vi "InjA-Image-RT.vi"() -> ()   [LabVIEW 2016]
uses:
  Controls/Cryo Readback.ctl
  Controls/Aperture states.ctl
  Controls/Faraday cup states.ctl
  Controls/GV states.ctl
  Controls/GP307 cluster.ctl
  <vilib>/userdefined/High Color/nirio_resource_hc.ctl
  PRIMELab-2017/Control/Common-Control/Glassman Control.ctl
  <vilib>/FPGAPlugInAG/cRIO-9074/niLvFpga_Open_cRIO-9074.vi
  <vilib>/Utility/error.llb/Error Cluster From Error Code.vi
  <vilib>/rvi/errors/niLvFpgaAdjustHostInterfaceError.vi
  <vilib>/functionblocks/Control/PID/PID.vi
  <vilib>/rvi/interface/nirviOpenFPGA/nirviOpenFPGA.xnode
  FPGA Bitfiles/Controlsoftware2_FPGATarget_InjFPGA_-aTnSXeY2bA.lvbitx
  InjA-Image-FPGA.vi
  <vilib>/rvi/interface/nirviReadWriteControl/nirviReadWriteControl.xnode
  <vilib>/functionblocks/FB Core/FB Core.xnode
  <vilib>/functionblocks/FB Property/FB Overlay DBL.ctl
  <vilib>/functionblocks/NI_FunctionBlock Libraries.lvlib
  NiFpgaLv.dll
  <vilib>/NI_Real-Time Target Support.lvlib
panel:
  in  "Tab Control":T1(tab)
  out "X-I":fxp<+/-,16,5>=1.28955078125
  out "X- V":fxp<+/-,16,5>=5.3388671875
  out "X+ I":fxp<+/-,16,5>=1.1064453125
  out "X+ V":fxp<+/-,16,5>=4.63671875
  out "Y+ V":fxp<+/-,16,5>=4.380859375
  out "Y+I":fxp<+/-,16,5>=1.068359375
  out "Y-V":fxp<+/-,16,5>=5.595703125
  out "Y-I":fxp<+/-,16,5>=1.36572265625
  out "Pre-acc V":fxp<+/-,16,5>=8.2509765625
  out "Pre-acc I":fxp<+/-,16,5>=2.544921875
  out "Einzel V":fxp<+/-,16,5>=7.4140625
  out "Einzel I":fxp<+/-,16,5>=1.6787109375
  out "X- Steerer Voltage Set":dbl
  out "X- Steerer HV Enable":bool
  out "X+ Steerer HV Enable":bool
  out "X+ Steerer Voltage Set":dbl
  out "Y- Steerer voltage set":dbl
  out "Y- Steerer HV Enable":bool
  out "Y+ Steerer HV Enable":bool
  out "Y+ Steerer voltage set":dbl
  out "Pre-Acc V set":dbl
  out "Pre-Acc HV Enable":bool
  out "Einzel HV Enable":bool
  out "Einzel V set":dbl
  in  "output low - injector":dbl
  in  "output high - injector":dbl=190.0
  out "Injector mag field set":dbl
  out "Injector mag field read 2":u8[](array[numeric])
  out "Injector mag field read":dbl
  out "Injector mag ps command":u8[](array[numeric])
  in  "derivative time (Td, min) - injector":dbl=0.01
  in  "integral time (Ti, min) - injector":dbl=0.01
  in  "proportional gain (Kc) - injector":dbl=10.0
  out "Injector mag command string":string
  out "Cryo Readback":T2
  out "Status":string
  out "On-time":string
  out "1st Stage Temp":string
  out "2nd Stage Temp":string
  out "Time since re-purge":string
  out "LowEnd Waist Vac Interlock":bool
  out "LowEnd Waist Vac Interlock bypass":bool
  out "Vac Interlock":bool
  out "Time since repurge":u8[](array[numeric])
  out "2nd stage temp":u8[](array[numeric])
  out "Cryo 1st stage temp":u8[](array[numeric])
  out "Cryo On-time":u8[](array[numeric])
  out "Cryo status":u8[](array[numeric])
  out "InjA Image Interlock bypass":bool
  out "Convectron 2":u8[](array[numeric])
  out "Ion Gauge 2":u8[](array[numeric])
  out "InjA Image Ion Gauge 1":dbl
  out "InjA Image Vac Cluster":T3
  out "InjA Image Convectron 1":dbl
  out "Convectron 1":u8[](array[numeric])
  out "Ion Gauge 1":u8[](array[numeric])
  out "Injector A Vac Interlock":bool
  out "Injector A Vac Interlock Bypass":bool
  out "Inj Image Aperture actuator":bool
  out "Inj Image FC actuator":bool
  out "Cryo Pump GV actuator":bool
  out "Beamline GV actuator":bool
  out "Inj Image Image  Aperture Position 2":T4
  out "Inj Image Image  Aperture Position":cluster{"IN sensor":bool, "OUT sensor":bool}
  out "Inj Image FC Status":T5
  out "Inj Image FC Position":cluster{"IN sensor":bool, "OUT sensor":bool}
  out "Beamline GV status":T6
  out "Beamline GV Position":T7
  out "Cryo Pump GV status":T6
  out "Cryo Pump GV Position":T7
  out "HV control loop error":errorcluster
  out "HV Readback loop error":errorcluster
  out "Injector Magnet error":errorcluster
  out "Cryo loop error":errorcluster
  out "GV Interlock loop error":errorcluster
  out "Acuator-Sensor loop error":errorcluster
  out "Vac cluster loop error":errorcluster
  out "Error Reporter":errorcluster
  in  "error in":errorcluster
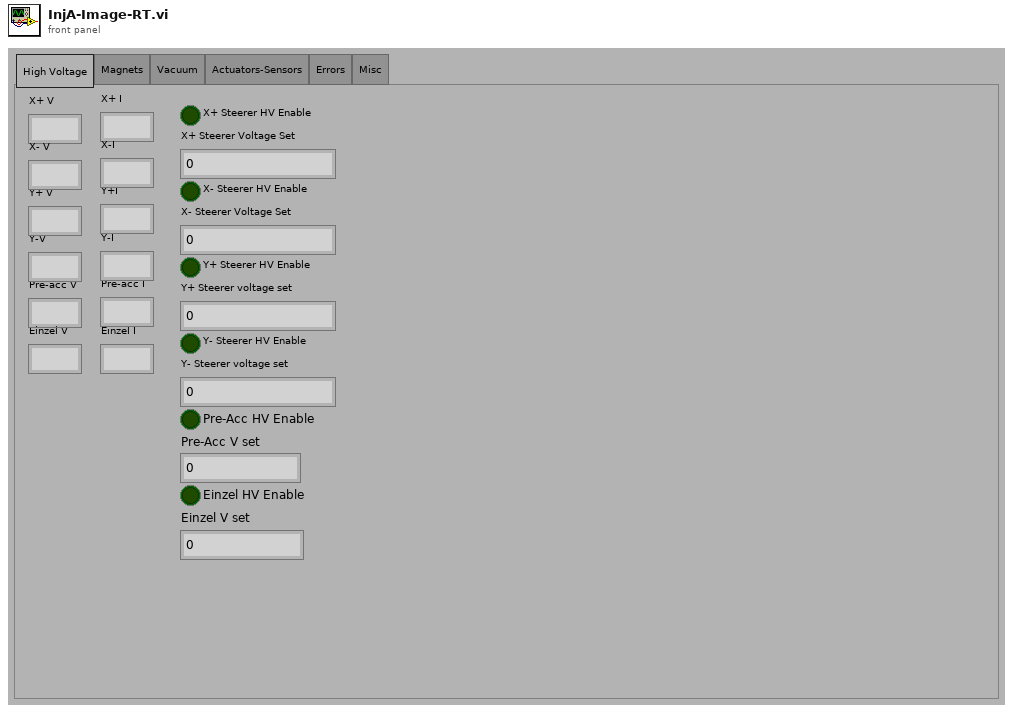
[diagram p1: front panel]
types:
  T1 = enum32{"High Voltage", "Magnets", "Vacuum", "Actuators-Sensors", "Errors", "Misc"}
  T2 = typedef "Cryo Readback.ctl" = cluster{"Status":string, "On-time":string, "1st Stage Temp":string, "2nd Stage Temp":string, "Time since re-purge":string}
  T3 = typedef "GP307 cluster.ctl" = cluster{"Ion gauge 1":string, "Convectron  Gauge 1 ":string, "Ion Gauge 2":string, "Convectrom Gauge 2":string}
  T4 = typedef "Aperture states.ctl" = enum16{"Aperture status unclear", "Aperture in", "Aperture out"}
  T5 = typedef "Faraday cup states.ctl" = enum16{"FC status unclear", "FC in", "FC out"}
  T6 = typedef "GV states.ctl" = enum16{"status unclear", "closed", "open"}
  T7 = cluster{"OPEN sensor":bool, "Closed sensor":bool}
  T8 = typedef "nirio_resource_hc.ctl" = tag
  T9 = cluster{"Stable 1":dbl, "Rare":dbl, "Stable 2":dbl}
  T10 = typedef "Glassman Control.ctl" = cluster{"V-program":fxp<+/-,16,5>, "HV Enable":bool}
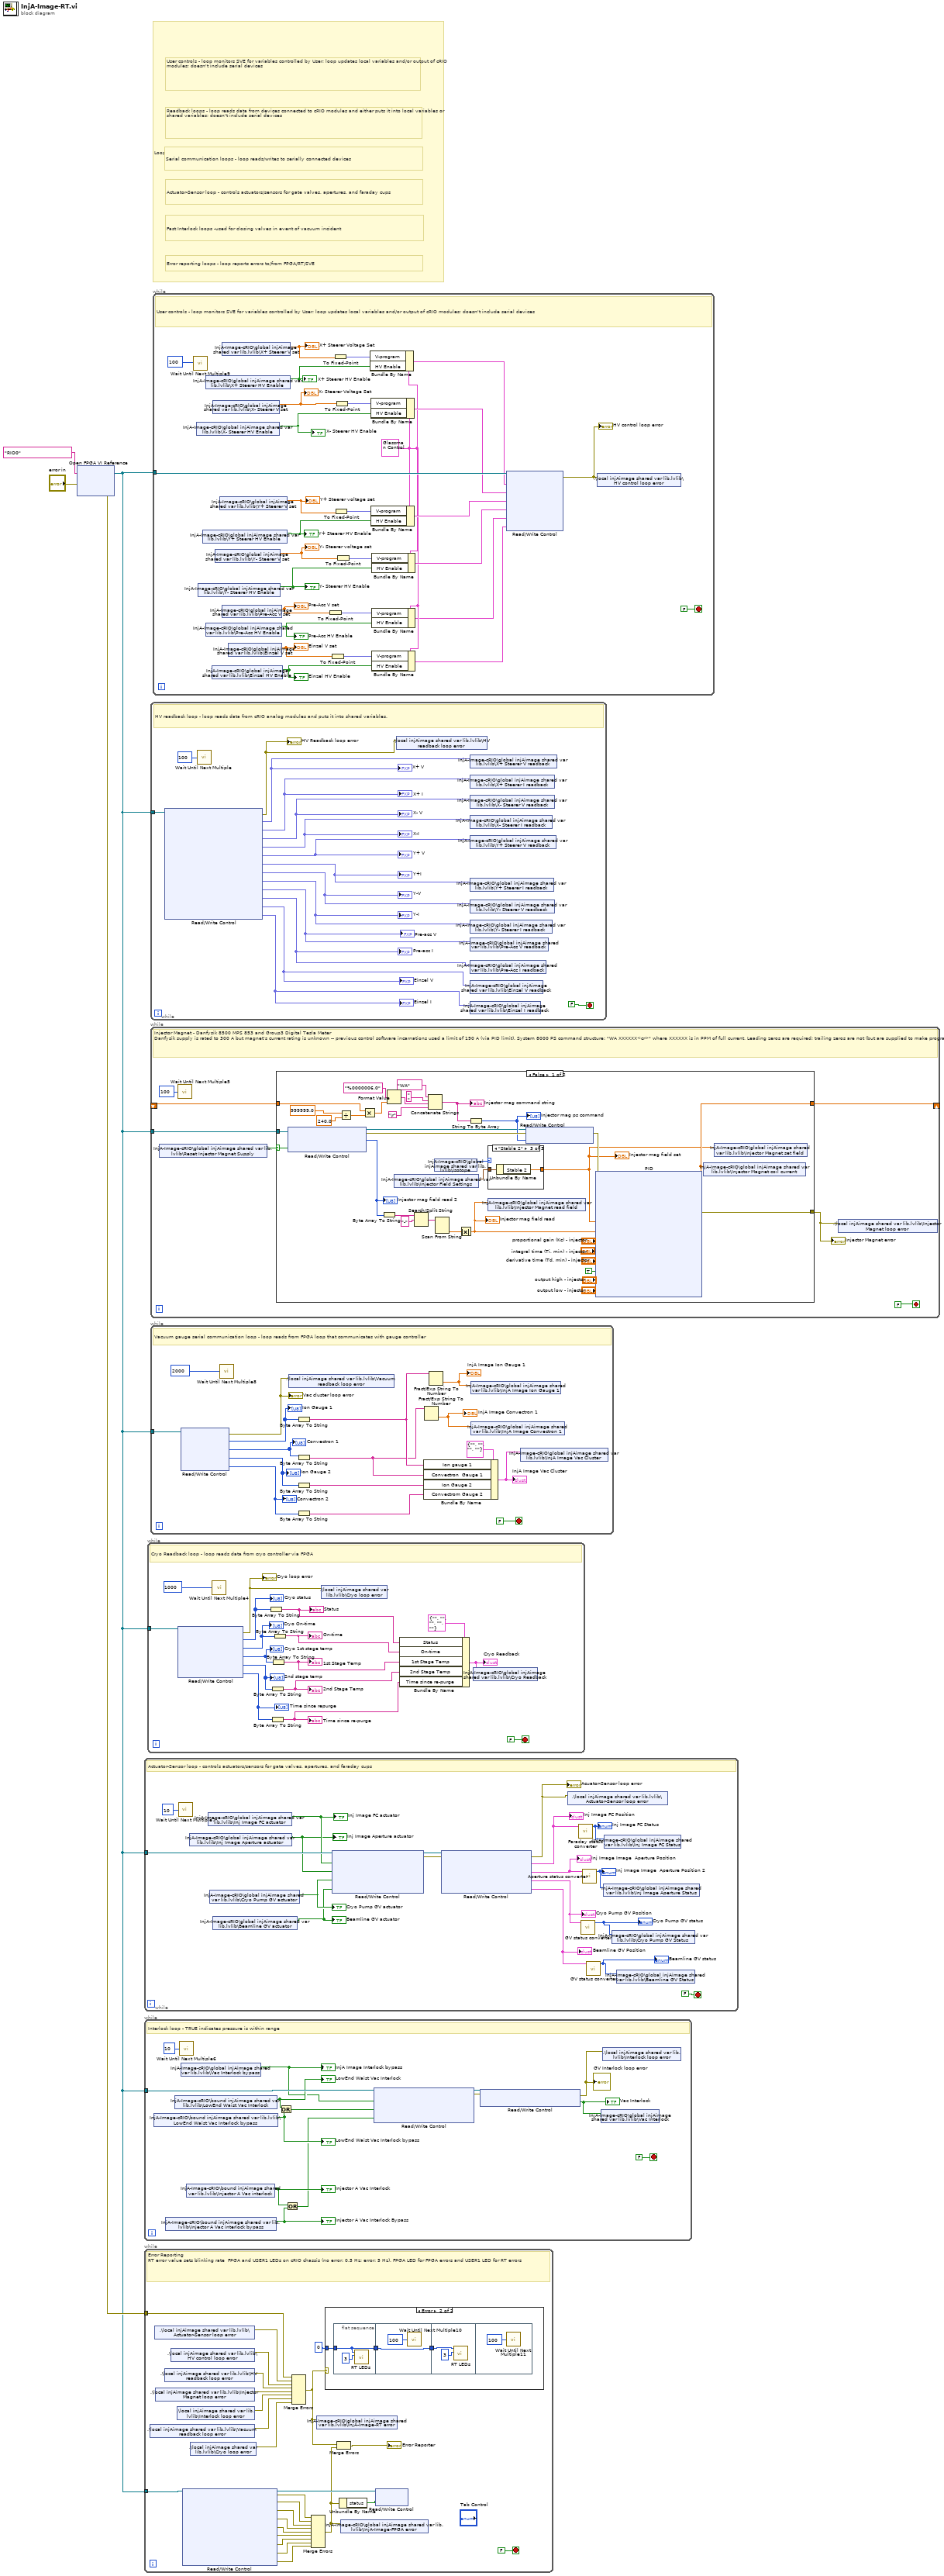
[diagram p0: block diagram]
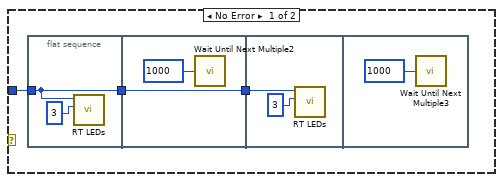
[diagram p2: hidden frame]
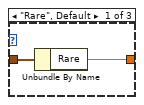
[diagram p3: hidden frame]
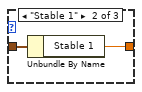
[diagram p4: hidden frame]
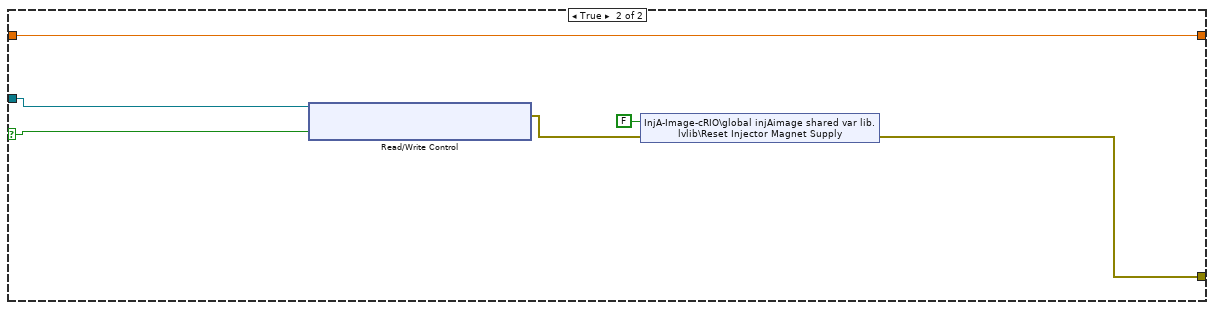
[diagram p5: hidden frame]
diagram:
  # "Serial communication loops - loop reads/writes to serially connected devices"
  # "Actuator-Sensor loop - controls actuators/sensors for gate valves, apertures, and faraday cups"
  # "Fast Interlock loops -used for closing valves in event of vacuum incident"
  # "Error reporting loops - loop reports errors to/from FPGA/RT/SVE"
  # "Readback loops - loop reads data from devices connected to cRIO modules and either puts it into local variables or shared variables; doesn't include serial devices"
  # "User controls - loop monitors SVE for variables controlled by User; loop updates local variables and/or output of cRIO modules; doesn't include serial devices"
  # "Loop legend - loops are color coded by responsibility"
  n1 = xnode "Open FPGA VI Reference"("error in"="error in", "resource name"=T8 "RIO0") -> ("FPGA VI Reference Out"=w1:refnum<k20>, "error out"=w2:errorcluster)
  n2 = while {
    tunnel: w1 -> [w22]
    stop <- FALSE stop-if-true
    # "Actuator-Sensor loop - controls actuators/sensors for gate valves, apertures, and faraday cups"
    n3 = call "Wait Until Next Multiple7"("Count(mSec)"=u32 10) -> ()  [unwired: 1 out]
    n4 = shared-variable "InjA-Image-cRIO\\global injAimage shared var lib.lvlib\\Inj Image Aperture actuator"() -> (w8:bool)  [unwired: 1 in, 1 out]
    "Inj Image Aperture actuator" <- w8
    n5 = shared-variable "InjA-Image-cRIO\\global injAimage shared var lib.lvlib\\Inj Image FC actuator"() -> (w9:bool)  [unwired: 1 in, 1 out]
    "Inj Image FC actuator" <- w9
    n6 = shared-variable "InjA-Image-cRIO\\global injAimage shared var lib.lvlib\\Cryo Pump GV actuator"() -> (w11:bool)  [unwired: 1 in, 1 out]
    "Cryo Pump GV actuator" <- w11
    n7 = shared-variable "InjA-Image-cRIO\\global injAimage shared var lib.lvlib\\Beamline GV actuator"() -> (w10:bool)  [unwired: 1 in, 1 out]
    "Beamline GV actuator" <- w10
    n8 = xnode "Read/Write Control"("FPGA VI Reference In"=w22, "Inj Image FC Actuator"=w9, "Inj Image Aperture Actuator"=w8, "Cryo Pump GV Actuator"=w11, "Beamline GV Actuator"=w10) -> ("FPGA VI Reference Out"=w20:refnum<k20>, "error out"=w18:errorcluster)  [unwired: 1 in]
    n9 = xnode "Read/Write Control"("FPGA VI Reference In"=w20, "error in"=w18) -> ("error out"=w12:errorcluster, "Inj Image FC Position"=w14:cluster{"IN sensor":bool, "OUT sensor":bool}, "Inj Image Aperture Position"=w13:cluster{"IN sensor":bool, "OUT sensor":bool}, "Cryo Pump GV Status"=w17:T7, "Beamline GV Status"=w16:T7)  [unwired: 1 out]
    "Cryo Pump GV Position" <- w17
    "Beamline GV Position" <- w16
    "Inj Image FC Position" <- w14
    "Inj Image Image  Aperture Position" <- w13
    "Acuator-Sensor loop error" <- w12
    n10 = shared-variable ".\\local injAimage shared var lib.lvlib\\Actuator-Sensor loop error"(w12) -> ()  [unwired: 1 in, 1 out]
    n11 = call "Faraday status converter.vi"("FC Position"=w14) -> ("FC Status"=w15:T5)  [unwired: 10 in]
    "Inj Image FC Status" <- w15
    n12 = call "GV status converter.vi"("Gate Valve"=w17) -> ("GV Status"=w6:T6)  [unwired: 10 in]
    "Cryo Pump GV status" <- w6
    n13 = call "Aperture status converter.vi"("Aperture Position"=w13) -> ("Aperture Status"=w5:T4)  [unwired: 10 in]
    "Inj Image Image  Aperture Position 2" <- w5
    n14 = call "GV status converter.vi"("Gate Valve"=w16) -> ("GV Status"=w7:T6)  [unwired: 10 in]
    "Beamline GV status" <- w7
    n15 = shared-variable "InjA-Image-cRIO\\global injAimage shared var lib.lvlib\\Inj Image Aperture Status"(w5) -> ()  [unwired: 1 in, 1 out]
    n16 = shared-variable "InjA-Image-cRIO\\global injAimage shared var lib.lvlib\\Inj Image FC Status"(w15) -> ()  [unwired: 1 in, 1 out]
    n17 = shared-variable "InjA-Image-cRIO\\global injAimage shared var lib.lvlib\\Cryo Pump GV Status"(w6) -> ()  [unwired: 1 in, 1 out]
    n18 = shared-variable "InjA-Image-cRIO\\global injAimage shared var lib.lvlib\\Beamline GV Status"(w7) -> ()  [unwired: 1 in, 1 out]
  }
  n19 = while {
    tunnel: w1 -> [w36]
    stop <- FALSE stop-if-true
    # "Interlock loop - TRUE indicates pressure is within range"
    n20 = shared-variable "InjA-Image-cRIO\\bound injAimage shared var lib.lvlib\\LowEnd Waist Vac Interlock bypass"() -> (w30:bool)  [unwired: 1 in, 1 out]
    "LowEnd Waist Vac Interlock bypass" <- w30
    n21 = shared-variable "InjA-Image-cRIO\\bound injAimage shared var lib.lvlib\\Injector A Vac interlock bypass"() -> (w25:bool)  [unwired: 1 in, 1 out]
    "Injector A Vac Interlock Bypass" <- w25
    n22 = shared-variable "InjA-Image-cRIO\\bound injAimage shared var lib.lvlib\\LowEnd Waist Vac Interlock"() -> (w28:bool)  [unwired: 1 in, 1 out]
    "LowEnd Waist Vac Interlock" <- w28
    n23 = call "Wait Until Next Multiple6"("Count(mSec)"=u32 10) -> ()  [unwired: 1 out]
    n24 = shared-variable "InjA-Image-cRIO\\global injAimage shared var lib.lvlib\\Vac Interlock bypass"() -> (w23:bool)  [unwired: 1 in, 1 out]
    "InjA Image Interlock bypass" <- w23
    n25 = shared-variable "InjA-Image-cRIO\\bound injAimage shared var lib.lvlib\\Injector A Vac interlock"() -> (w26:bool)  [unwired: 1 in, 1 out]
    "Injector A Vac Interlock" <- w26
    n26 = Or(x=w28, y=w30) -> (x .or. y?=w29:bool)
    n27 = Or(x=w26, y=w25) -> (x .or. y?=w24:bool)
    n28 = xnode "Read/Write Control"("FPGA VI Reference In"=w36, "Vac Interlock Bypass"=w23, "LowEnd Waist Vac Interlock"=w29, "InjectorA Vac Interlock"=w24) -> ("FPGA VI Reference Out"=w35:refnum<k20>, "error out"=w34:errorcluster)  [unwired: 1 in]
    n29 = xnode "Read/Write Control"("FPGA VI Reference In"=w35, "error in"=w34) -> ("error out"=w33:errorcluster, "Vac Interlock"=w27:bool)  [unwired: 1 out]
    "GV Interlock loop error" <- w33
    "Vac Interlock" <- w27
    n30 = shared-variable "InjA-Image-cRIO\\global injAimage shared var lib.lvlib\\Vac Interlock"(w27) -> ()  [unwired: 1 in, 1 out]
    n31 = shared-variable ".\\local injAimage shared var lib.lvlib\\Interlock loop error"(w33) -> ()  [unwired: 1 in, 1 out]
  }
  n32 = while {
    tunnel: w1 -> [w60]
    tunnel: w2 -> [w44]
    stop <- FALSE stop-if-true
    # "Error Reporting\nRT error value sets blinking rate  FPGA and USER1 LEDs on cRIO chassis (no error: 0.5 Hz; error: 5 Hz). FPGA LED for FPGA errors and USER1 LED for RT errors"
    n33 = shared-variable ".\\local injAimage shared var lib.lvlib\\Vacuum readback loop error"() -> (w46:errorcluster)  [unwired: 1 in, 1 out]
    n34 = shared-variable ".\\local injAimage shared var lib.lvlib\\Actuator-Sensor loop error"() -> (w43:errorcluster)  [unwired: 1 in, 1 out]
    n35 = shared-variable ".\\local injAimage shared var lib.lvlib\\Injector Magnet loop error"() -> (w48:errorcluster)  [unwired: 1 in, 1 out]
    n36 = shared-variable ".\\local injAimage shared var lib.lvlib\\HV readback loop error"() -> (w49:errorcluster)  [unwired: 1 in, 1 out]
    n37 = shared-variable ".\\local injAimage shared var lib.lvlib\\HV control loop error"() -> (w42:errorcluster)  [unwired: 1 in, 1 out]
    n38 = shared-variable ".\\local injAimage shared var lib.lvlib\\Interlock loop error"() -> (w47:errorcluster)  [unwired: 1 in, 1 out]
    n39 = xnode "Read/Write Control"("FPGA VI Reference In"=w60) -> ("FPGA VI Reference Out"=w59:refnum<k20>, "error out"=w37:errorcluster, "GV Interlock loop error"=w58:errorcluster, "Actuator-Sensor Loop error"=w57:errorcluster, "Injector Hall Probe error"=w56:errorcluster, "Injector Magnet control error"=w55:errorcluster, "Vac readback loop error"=w54:errorcluster, "HV control loop error"=w53:errorcluster, "Cryo pump error"=w51:errorcluster, "HV Readback loop"=w50:errorcluster)  [unwired: 1 in]
    n40 = shared-variable ".\\local injAimage shared var lib.lvlib\\Cryo loop error"() -> (w45:errorcluster)  [unwired: 1 in, 1 out]
    n41 = Merge Errors(w44, w43, w42, w49, w48, w47, w46, w45) -> (w38:errorcluster)
    n42 = Merge Errors(w37, w58, w57, w56, w55, w54, w53, w51, w50) -> (w40:errorcluster)
    n43 = shared-variable "InjA-Image-cRIO\\global injAimage shared var lib.lvlib\\InjA-Image-RT error"(w38) -> ()  [unwired: 1 in, 1 out]
    n44 = case shown="Error" w38 {
      tunnel: 0 -> [w64 w72]
      frame No Error {
        n45 = flat-sequence {
          tunnel: w64 -> [w65]
          tunnel: [w65] -> w62
          tunnel: [w67] -> w63
          tunnel: w62 -> [w67]
          tunnel: w63 -> [w69]
          frame #0 {
            n46 = call <vilib>:"RT LEDs.vi"("State"=3, "LED Num"=w65) -> ()  [unwired: 4 in, 2 out]
          }
          frame #1 {
            n47 = call "Wait Until Next Multiple2"("Count(mSec)"=u16 1000) -> ()  [unwired: 1 out]
          }
          frame #2 {
            n48 = call <vilib>:"RT LEDs.vi"("State"=3, "LED Num"=w69) -> ()  [unwired: 4 in, 2 out]
          }
          frame #3 {
            n49 = call "Wait Until Next Multiple3"("Count(mSec)"=u16 1000) -> ()  [unwired: 1 out]
          }
        }
      }
      frame Error {
        n50 = flat-sequence {
          tunnel: [w75] -> w74
          tunnel: w72 -> [w75]
          tunnel: w74 -> [w77]
          tunnel: [w77] -> w73
          tunnel: w73 -> [w79]
          frame #0 {
            n51 = call <vilib>:"RT LEDs.vi"("State"=3, "LED Num"=w75) -> ()  [unwired: 4 in, 2 out]
          }
          frame #1 {
            n52 = call "Wait Until Next Multiple10"("Count(mSec)"=u16 100) -> ()  [unwired: 1 out]
          }
          frame #2 {
            n53 = call <vilib>:"RT LEDs.vi"("State"=3, "LED Num"=w79) -> ()  [unwired: 4 in, 2 out]
          }
          frame #3 {
            n54 = call "Wait Until Next Multiple11"("Count(mSec)"=u16 100) -> ()  [unwired: 1 out]
          }
        }
      }
    }
    n55 = Merge Errors(w38, w40) -> (→"Error Reporter":errorcluster)
    n56 = Unbundle By Name(w40) -> ("status"=w61:bool)
    n57 = shared-variable "InjA-Image-cRIO\\global injAimage shared var lib.lvlib\\InjA-Image-FPGA error"(w40) -> ()  [unwired: 1 in, 1 out]
    n58 = xnode "Read/Write Control"("FPGA VI Reference In"=w59, "RT error"=w61) -> ()  [unwired: 1 in, 2 out]
  }
  n59 = while {
    tunnel: w1 -> [w96]
    stop <- FALSE stop-if-true
    # "Cryo Readback loop - loop reads data from cryo controller via FPGA"
    n60 = xnode "Read/Write Control"("FPGA VI Reference In"=w96) -> ("error out"=w82:errorcluster, "Cryo status"=w93:u8[], "Cryo On-time"=w94:u8[], "1st stage temp"=w95:u8[], "2nd stage temp"=w92:u8[], "Time since repurge"=w91:u8[])  [unwired: 1 in, 1 out]
    "Cryo status" <- w93
    "Cryo On-time" <- w94
    "Cryo 1st stage temp" <- w95
    "Cryo loop error" <- w82
    "2nd stage temp" <- w92
    "Time since repurge" <- w91
    n61 = call "Wait Until Next Multiple4"("Count(mSec)"=u32 1000 ("millisecond multiple")) -> ()  [unwired: 1 out]
    n62 = Byte Array To String(unsigned byte array=w93) -> (string=w87:string)
    "Status" <- w87
    n63 = Byte Array To String(unsigned byte array=w92) -> (string=w84:string)
    "2nd Stage Temp" <- w84
    n64 = Byte Array To String(unsigned byte array=w91) -> (string=w83:string)
    "Time since re-purge" <- w83
    n65 = Byte Array To String(unsigned byte array=w95) -> (string=w85:string)
    "1st Stage Temp" <- w85
    n66 = Byte Array To String(unsigned byte array=w94) -> (string=w86:string)
    "On-time" <- w86
    n67 = shared-variable ".\\local injAimage shared var lib.lvlib\\Cryo loop error"(w82) -> ()  [unwired: 1 in, 1 out]
    n68 = Bundle By Name(cluster=T2 {"Status"="", "On-time"="", "1st Stage Temp"="", "2nd Stage Temp"="", "Time since re-purge"=""} ("Cryo Readback"), "Status"=w87, "On-time"=w86, "1st Stage Temp"=w85, "2nd Stage Temp"=w84, "Time since re-purge"=w83) -> (w89:T2)
    "Cryo Readback" <- w89
    n69 = shared-variable "InjA-Image-cRIO\\global injAimage shared var lib.lvlib\\Cryo Readback"(w89) -> ()  [unwired: 1 in, 1 out]
  }
  n70 = while {
    shift-right: [w100] -> _
    shift-left: _ -> [w102]
    tunnel: w1 -> [w103]
    stop <- FALSE stop-if-true
    # "Injector Magnet - Danfysik 8500 MPS 853 and Group3 Digital Tesla Meter\nDanfysik supply is rated to 300 A but magnet's current rating is unknown -- previous control software incarnations used a limit of 190 A (via PID limit). System 8000 PS command structure: \"WA XXXXXX<cr>\" where XXXXXX is in PPM of full current. Leading zeros are required; trailing zeros are not (but are supplied to make programming easier)"
    n71 = shared-variable "InjA-Image-cRIO\\global injAimage shared var lib.lvlib\\Reset Injector Magnet Supply"() -> (w99:bool)  [unwired: 1 in, 1 out]
    n72 = call "Wait Until Next Multiple5"("Count(mSec)"=u32 100 ("millisecond multiple")) -> ()  [unwired: 1 out]
    n73 = case shown="False" w99 {
      selector: w99 -> [w110 w214]
      tunnel: w103 -> [w125 w216]
      tunnel: w102 -> [w121 w215]
      tunnel: [w111 w215] -> w100
      tunnel: [w109 w211] -> w98
      frame False {
        n74 = xnode "Read/Write Control"("FPGA VI Reference In"=w125, "Inj Magnet Reset"=w110) -> ("FPGA VI Reference Out"=w119:refnum<k20>, "error out"=w124:errorcluster, "Injector Mag Field read"=w120:u8[])  [unwired: 1 in]
        "Injector mag field read 2" <- w120
        n75 = Divide(x=999999.0 ("y"), y=240.0) -> (x/y=w113:dbl)
        n76 = Multiply(x=w121, y=w113) -> (x*y=w134:dbl)
        n77 = Byte Array To String(unsigned byte array=w120) -> (string=w131:string)
        n78 = Format Value(format string="%0000006.0", value (0)=w134) -> (output string=w137:string)  [unwired: 1 out]
        n79 = shared-variable "InjA-Image-cRIO\\global injAimage shared var lib.lvlib\\Injector Field Settings"() -> (w105:T9)  [unwired: 1 in, 1 out]
        n80 = Search/Split String(string=w131, search string/char (-)="-") -> (match + rest of string=w122:string)  [unwired: 3 out]
        n81 = Concatenate Strings("WA", " ", w137, "\r") -> (w138:string)
        "Injector mag command string" <- w138
        n82 = shared-variable "InjA-Image-cRIO\\global injAimage shared var lib.lvlib\\Isotope"() -> (w107:enum16{"Rare", "Stable 1", "Stable 2"})  [unwired: 1 in, 1 out]
        n83 = Scan From String(input string=w122) -> (output 1=w130:dbl)  [unwired: 3 in, 4 out]
        n84 = Absolute Value(x=w130) -> (abs(x)=w108:dbl)
        "Injector mag field read" <- w108
        n85 = String To Byte Array(string=w138) -> (unsigned byte array=w123:u8[])
        "Injector mag ps command" <- w123
        n86 = case shown="\"Stable 2\"" w107 {
          tunnel: w105 -> [w139 w142 w144]
          tunnel: [w140 w141 w143] -> w106
          frame "Rare", Default {
            n87 = Unbundle By Name(w139) -> ("Rare"=w140:dbl)
          }
          frame "Stable 1" {
            n88 = Unbundle By Name(w142) -> ("Stable 1"=w141:dbl)
          }
          frame "Stable 2" {
            n89 = Unbundle By Name(w144) -> ("Stable 2"=w143:dbl)
          }
        }
        "Injector mag field set" <- w106
        n90 = shared-variable "InjA-Image-cRIO\\global injAimage shared var lib.lvlib\\Injector Magnet read field"(w108) -> ()  [unwired: 1 in, 1 out]
        n91 = xnode "Read/Write Control"("FPGA VI Reference In"=w119, "error in"=w124, "Injector Magnet Set"=w123) -> ("error out"=w118:errorcluster)  [unwired: 1 out]
        n92 = xnode "PID"("error in"=w118, "setpoint"=w106, "process variable"=w108, "proportional gain (Kc)"="proportional gain (Kc) - injector", "integral time (Ti, min)"="integral time (Ti, min) - injector", "derivative time (Td, min)"="derivative time (Td, min) - injector", "auto? (T)"=TRUE, "output high"="output high - injector", "output low"="output low - injector") -> ("error out"=w109:errorcluster, "output"=w111:dbl)
        n93 = shared-variable "InjA-Image-cRIO\\global injAimage shared var lib.lvlib\\Injector Magnet coil current"(w111) -> ()  [unwired: 1 in, 1 out]
        n94 = shared-variable "InjA-Image-cRIO\\global injAimage shared var lib.lvlib\\Injector Magnet set field"(w106) -> ()  [unwired: 1 in, 1 out]
      }
      frame True {
        n95 = xnode "Read/Write Control"("FPGA VI Reference In"=w216, "Inj Magnet Reset"=w214) -> ("error out"=w212:errorcluster)  [unwired: 1 in, 1 out]
        n96 = shared-variable "InjA-Image-cRIO\\global injAimage shared var lib.lvlib\\Reset Injector Magnet Supply"(FALSE ("Reset Injector Magnet Supply"), error in=w212) -> (error out=w211:errorcluster)
      }
    }
    "Injector Magnet error" <- w98
    n97 = shared-variable ".\\local injAimage shared var lib.lvlib\\Injector Magnet loop error"(w98) -> ()  [unwired: 1 in, 1 out]
  }
  n98 = while {
    tunnel: w1 -> [w227]
    stop <- FALSE stop-if-true
    # "Vacuum gauge serial communication loop - loop reads from FPGA loop that communicates with gauge controller"
    n99 = xnode "Read/Write Control"("FPGA VI Reference In"=w227) -> ("error out"=w222:errorcluster, "Ion gauge 1"=w228:u8[], "Convectron 1"=w224:u8[], "Ion gauge 2"=w229:u8[], "Convectron 2"=w230:u8[])  [unwired: 1 in, 1 out]
    "Ion Gauge 1" <- w228
    "Convectron 1" <- w224
    "Ion Gauge 2" <- w229
    "Convectron 2" <- w230
    "Vac cluster loop error" <- w222
    n100 = call "Wait Until Next Multiple8"("Count(mSec)"=u32 2000 ("millisecond multiple")) -> ()  [unwired: 1 out]
    n101 = shared-variable ".\\local injAimage shared var lib.lvlib\\Vacuum readback loop error"(w222) -> ()  [unwired: 1 in, 1 out]
    n102 = Byte Array To String(unsigned byte array=w228) -> (string=w225:string)
    n103 = Byte Array To String(unsigned byte array=w224) -> (string=w223:string)
    n104 = Byte Array To String(unsigned byte array=w229) -> (string=w231:string)
    n105 = Byte Array To String(unsigned byte array=w230) -> (string=w232:string)
    n106 = Bundle By Name(cluster=T3 {"Ion gauge 1"="", "Convectron  Gauge 1 "="", "Ion Gauge 2"="", "Convectrom Gauge 2"=""} ("Ion gauge cluster control"), "Ion gauge 1"=w225, "Convectron  Gauge 1"=w223, "Ion Gauge 2"=w231, "Convectrom Gauge 2"=w232) -> (w219:T3)
    "InjA Image Vac Cluster" <- w219
    n107 = Fract/Exp String To Number(string=w223) -> (number=w218:dbl)  [unwired: 3 in, 1 out]
    "InjA Image Convectron 1" <- w218
    n108 = Fract/Exp String To Number(string=w225) -> (number=w217:dbl)  [unwired: 3 in, 1 out]
    "InjA Image Ion Gauge 1" <- w217
    n109 = shared-variable "InjA-Image-cRIO\\global injAimage shared var lib.lvlib\\InjA Image Ion Gauge 1"(w217) -> ()  [unwired: 1 in, 1 out]
    n110 = shared-variable "InjA-Image-cRIO\\global injAimage shared var lib.lvlib\\InjA Image Convectron 1"(w218) -> ()  [unwired: 1 in, 1 out]
    n111 = shared-variable "InjA-Image-cRIO\\global injAimage shared var lib.lvlib\\InjA Image Vac Cluster"(w219) -> ()  [unwired: 1 in, 1 out]
  }
  n112 = while {
    tunnel: w1 -> [w234]
    stop <- FALSE stop-if-true
    # "HV readback loop - loop reads data from cRIO analog modules and puts it into shared variables."
    n113 = xnode "Read/Write Control"("FPGA VI Reference In"=w234) -> ("error out"=w233:errorcluster, "X+ Steerer Monitor.I-monitor"=w246:fxp<+/-,16,5>, "X+ Steerer Monitor.V-monitor"=w245:fxp<+/-,16,5>, "X- Steerer Monitor.I-monitor"=w244:fxp<+/-,16,5>, "X- Steerer Monitor.V-monitor"=w243:fxp<+/-,16,5>, "Y+ Steerer Monitor.I-monitor"=w242:fxp<+/-,16,5>, "Y+ Steerer Monitor.V-monitor"=w235:fxp<+/-,16,5>, "Y- Steerer Monitor.I-monitor"=w236:fxp<+/-,16,5>, "Y- Steerer Monitor.V-monitor"=w237:fxp<+/-,16,5>, "Pre-Acc Monitor.I-monitor"=w238:fxp<+/-,16,5>, "Pre-Acc Monitor.V-monitor"=w239:fxp<+/-,16,5>, "Einzel Monitor.I-monitor"=w240:fxp<+/-,16,5>, "Einzel Monitor.V-monitor"=w241:fxp<+/-,16,5>)  [unwired: 1 in, 1 out]
    "Y+ V" <- w242
    "Y+I" <- w235
    "Y-V" <- w236
    "Y-I" <- w237
    "Pre-acc V" <- w238
    "Pre-acc I" <- w239
    "Einzel V" <- w240
    "Einzel I" <- w241
    "X+ V" <- w246
    "X+ I" <- w245
    "X- V" <- w244
    "X-I" <- w243
    "HV Readback loop error" <- w233
    n114 = call "Wait Until Next Multiple"("Count(mSec)"=u32 100) -> ()  [unwired: 1 out]
    n115 = shared-variable ".\\local injAimage shared var lib.lvlib\\HV readback loop error"(w233) -> ()  [unwired: 1 in, 1 out]
    n116 = shared-variable "InjA-Image-cRIO\\global injAimage shared var lib.lvlib\\X+ Steerer V readback"(w246) -> ()  [unwired: 1 in, 1 out]
    n117 = shared-variable "InjA-Image-cRIO\\global injAimage shared var lib.lvlib\\X+ Steerer I readback"(w245) -> ()  [unwired: 1 in, 1 out]
    n118 = shared-variable "InjA-Image-cRIO\\global injAimage shared var lib.lvlib\\X- Steerer V readback"(w244) -> ()  [unwired: 1 in, 1 out]
    n119 = shared-variable "InjA-Image-cRIO\\global injAimage shared var lib.lvlib\\X- Steerer I readback"(w243) -> ()  [unwired: 1 in, 1 out]
    n120 = shared-variable "InjA-Image-cRIO\\global injAimage shared var lib.lvlib\\Y+ Steerer V readback"(w242) -> ()  [unwired: 1 in, 1 out]
    n121 = shared-variable "InjA-Image-cRIO\\global injAimage shared var lib.lvlib\\Y+ Steerer I readback"(w235) -> ()  [unwired: 1 in, 1 out]
    n122 = shared-variable "InjA-Image-cRIO\\global injAimage shared var lib.lvlib\\Y- Steerer V readback"(w236) -> ()  [unwired: 1 in, 1 out]
    n123 = shared-variable "InjA-Image-cRIO\\global injAimage shared var lib.lvlib\\Y- Steerer I readback"(w237) -> ()  [unwired: 1 in, 1 out]
    n124 = shared-variable "InjA-Image-cRIO\\global injAimage shared var lib.lvlib\\Pre-Acc V readback"(w238) -> ()  [unwired: 1 in, 1 out]
    n125 = shared-variable "InjA-Image-cRIO\\global injAimage shared var lib.lvlib\\Pre-Acc I readback"(w239) -> ()  [unwired: 1 in, 1 out]
    n126 = shared-variable "InjA-Image-cRIO\\global injAimage shared var lib.lvlib\\Einzel V readback"(w240) -> ()  [unwired: 1 in, 1 out]
    n127 = shared-variable "InjA-Image-cRIO\\global injAimage shared var lib.lvlib\\Einzel I readback"(w241) -> ()  [unwired: 1 in, 1 out]
  }
  n128 = while {
    tunnel: w1 -> [w277]
    stop <- FALSE stop-if-true
    w257 = T10 {"V-program"=0.0, "HV Enable"=FALSE} ("Glassman Control")
    # "User controls - loop monitors SVE for variables controlled by User; loop updates local variables and/or output of cRIO modules; doesn't include serial devices"
    n129 = call "Wait Until Next Multiple9"("Count(mSec)"=u32 100 ("millisecond multiple")) -> ()  [unwired: 1 out]
    n130 = shared-variable "InjA-Image-cRIO\\global injAimage shared var lib.lvlib\\X- Steerer HV Enable"() -> (w263:bool)  [unwired: 1 in, 1 out]
    "X- Steerer HV Enable" <- w263
    n131 = shared-variable "InjA-Image-cRIO\\global injAimage shared var lib.lvlib\\Y- Steerer HV Enable"() -> (w259:bool)  [unwired: 1 in, 1 out]
    "Y- Steerer HV Enable" <- w259
    n132 = shared-variable "InjA-Image-cRIO\\global injAimage shared var lib.lvlib\\Y+ Steerer HV Enable"() -> (w261:bool)  [unwired: 1 in, 1 out]
    "Y+ Steerer HV Enable" <- w261
    n133 = shared-variable "InjA-Image-cRIO\\global injAimage shared var lib.lvlib\\X+ Steerer HV Enable"() -> (w266:bool)  [unwired: 1 in, 1 out]
    "X+ Steerer HV Enable" <- w266
    n134 = shared-variable "InjA-Image-cRIO\\global injAimage shared var lib.lvlib\\Pre-Acc HV Enable"() -> (w251:bool)  [unwired: 1 in, 1 out]
    "Pre-Acc HV Enable" <- w251
    n135 = shared-variable "InjA-Image-cRIO\\global injAimage shared var lib.lvlib\\Einzel HV Enable"() -> (w253:bool)  [unwired: 1 in, 1 out]
    "Einzel HV Enable" <- w253
    n136 = shared-variable "InjA-Image-cRIO\\global injAimage shared var lib.lvlib\\X- Steerer V set"() -> (w264:dbl)  [unwired: 1 in, 1 out]
    "X- Steerer Voltage Set" <- w264
    n137 = shared-variable "InjA-Image-cRIO\\global injAimage shared var lib.lvlib\\Y- Steerer V set"() -> (w260:dbl)  [unwired: 1 in, 1 out]
    "Y- Steerer voltage set" <- w260
    n138 = shared-variable "InjA-Image-cRIO\\global injAimage shared var lib.lvlib\\Y+ Steerer V set"() -> (w262:dbl)  [unwired: 1 in, 1 out]
    "Y+ Steerer voltage set" <- w262
    n139 = shared-variable "InjA-Image-cRIO\\global injAimage shared var lib.lvlib\\X+ Steerer V set"() -> (w265:dbl)  [unwired: 1 in, 1 out]
    "X+ Steerer Voltage Set" <- w265
    n140 = shared-variable "InjA-Image-cRIO\\global injAimage shared var lib.lvlib\\Pre-Acc V set"() -> (w252:dbl)  [unwired: 1 in, 1 out]
    "Pre-Acc V set" <- w252
    n141 = shared-variable "InjA-Image-cRIO\\global injAimage shared var lib.lvlib\\Einzel V set"() -> (w254:dbl)  [unwired: 1 in, 1 out]
    "Einzel V set" <- w254
    n142 = To Fixed-Point(number=w252) -> (fixed-point=w250:fxp<+/-,16,5>)  [unwired: 1 in]
    n143 = To Fixed-Point(number=w254) -> (fixed-point=w249:fxp<+/-,16,5>)  [unwired: 1 in]
    n144 = To Fixed-Point(number=w265) -> (fixed-point=w270:fxp<+/-,20,5>)  [unwired: 1 in]
    n145 = To Fixed-Point(number=w262) -> (fixed-point=w274:fxp<+/-,16,5>)  [unwired: 1 in]
    n146 = To Fixed-Point(number=w264) -> (fixed-point=w269:fxp<+/-,16,5>)  [unwired: 1 in]
    n147 = To Fixed-Point(number=w260) -> (fixed-point=w273:fxp<+/-,16,5>)  [unwired: 1 in]
    n148 = Bundle By Name(cluster=w257, "V-program"=w270, "HV Enable"=w266) -> (w267:T10)
    n149 = Bundle By Name(cluster=w257, "V-program"=w269, "HV Enable"=w263) -> (w268:T10)
    n150 = Bundle By Name(cluster=w257, "V-program"=w274, "HV Enable"=w261) -> (w271:T10)
    n151 = Bundle By Name(cluster=w257, "V-program"=w273, "HV Enable"=w259) -> (w272:T10)
    n152 = Bundle By Name(cluster=w257, "V-program"=w250, "HV Enable"=w251) -> (w256:T10)
    n153 = Bundle By Name(cluster=w257, "V-program"=w249, "HV Enable"=w253) -> (w255:T10)
    n154 = xnode "Read/Write Control"("FPGA VI Reference In"=w277, "X+ Steerer V set"=w267, "X- Steerer V set"=w268, "Y+ Steerer V set"=w271, "Y- Steerer V set"=w272, "Pre-Acc V set"=w256, "Einzel V set"=w255) -> ("error out"=w275:errorcluster)  [unwired: 1 in, 1 out]
    "HV control loop error" <- w275
    n155 = shared-variable ".\\local injAimage shared var lib.lvlib\\HV control loop error"(w275) -> ()  [unwired: 1 in, 1 out]
  }
